vi "from string array.vi"(8 "error in (no error)":errorcluster, 9 "String Array":string[][](array[string]), 10 "version":string, 11 "Multiplexer configuration in":refnum<class "Multiplexer configuration.lvclass">) -> (0 "error out":errorcluster, 3 "Multiplexer configuration out":refnum<class "Multiplexer configuration.lvclass">)   [LabVIEW 2021, in "Multiplexer configuration.lvclass"]
uses:
  Multiplexer configuration.lvclass
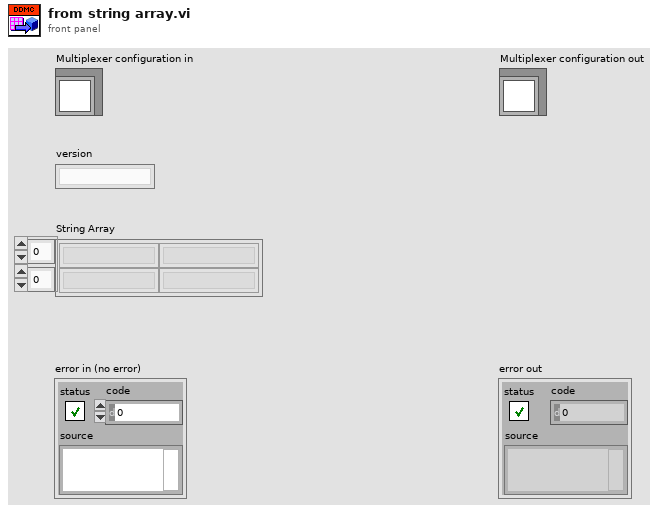
[diagram p1: front panel]
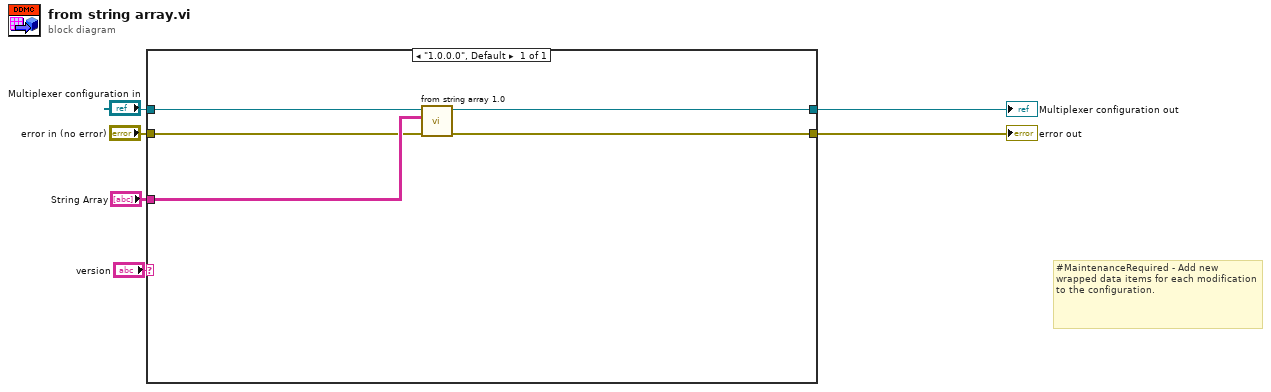
[diagram p0: block diagram]
diagram:
  # "#MaintenanceRequired - Add new wrapped data items for each modification to the configuration."
  n1 = case shown="\"1.0.0.0\", Default" "version" {
    tunnel: "String Array" -> [w11]
    tunnel: "Multiplexer configuration in" -> [w10]
    tunnel: "error in (no error)" -> [w9]
    tunnel: [w8] -> w2
    tunnel: [w7] -> w1
    frame "1.0.0.0", Default {
      n2 = call "from string array 1.0.vi"("error in (no error)"=w9, "String Array"=w11, "Multiplexer configuration in"=w10) -> ("error out"=w7:errorcluster, "Multiplexer configuration out"=w8:refnum<class "Multiplexer configuration.lvclass">)  [unwired: 7 in]
    }
  }
  "error out" <- w1
  "Multiplexer configuration out" <- w2
